vi "step7 SolveUpperRightCorner.vi"(11 "cube in":T1) -> (3 "cube out":T1)   [LabVIEW 2011]
uses:
  Typedef/cube.ctl
  Typedef/face.ctl
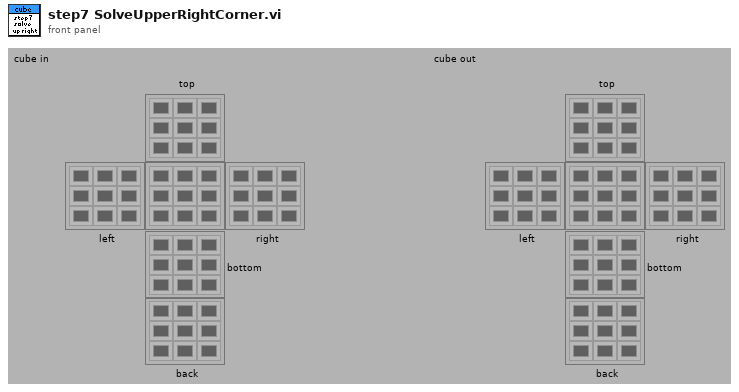
[diagram p1: front panel]
types:
  T1 = typedef "cube.ctl" = cluster{"top":T2, "left":T2, "right":T2, "bottom":T2, "back":T2, "front":T2}
  T2 = typedef "face.ctl" = u32[][]
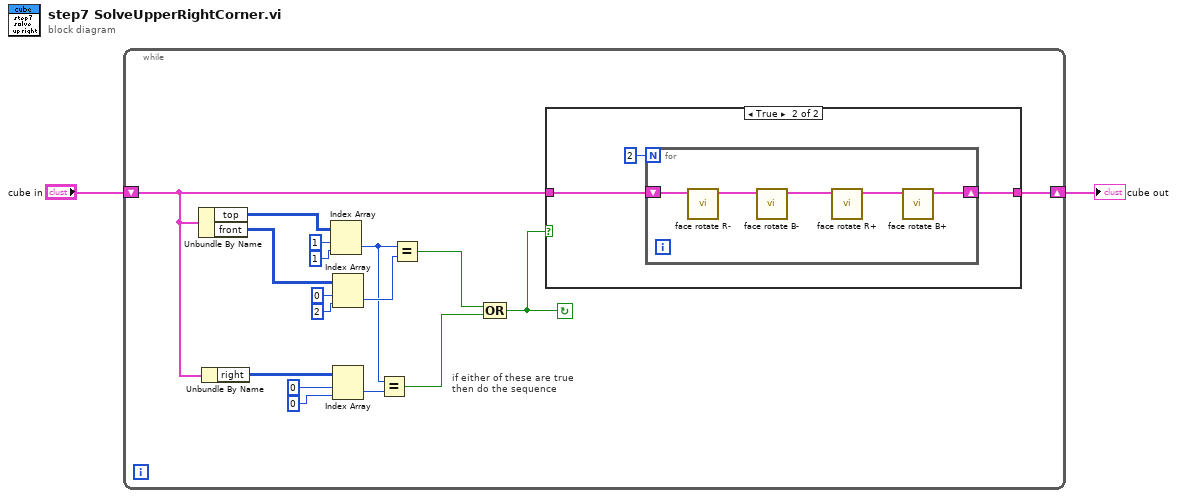
[diagram p0: block diagram]
diagram:
  n1 = while {
    shift-right: [w11] -> w1
    shift-left: "cube in" -> [w12]
    stop <- w10 continue-if-true
    # "if either of these are true\nthen do the sequence"
    n2 = Unbundle By Name(w12) -> ("top"=w9:T2, "front"=w6:T2)
    n3 = Unbundle By Name(w12) -> ("right"=w17:T2)
    n4 = Index Array(array=w9, index (row)=1, index (col)=1 ("disabled index (col)")) -> (element=w3:u32)
    n5 = Index Array(array=w6, index (row)=0, index (col)=2 ("disabled index (col)")) -> (element=w5:u32)
    n6 = Index Array(array=w17, index (row)=0, index (col)=0 ("disabled index (col)")) -> (element=w4:u32)
    n7 = Equal?(x=w3, y=w4) -> (x = y?=w13:bool)
    n8 = Equal?(x=w3, y=w5) -> (x = y?=w14:bool)
    n9 = Compound Arithmetic op=OR(w14, w13) -> (w10:bool)
    n10 = case shown="True" w10 {
      tunnel: w12 -> [w20 w23]
      tunnel: [w20 w22] -> w11
      frame False {
      }
      frame True {
        n11 = for {
          N: 2 -> [_]
          shift-right: [w24] -> w22
          shift-left: w23 -> [w28]
          n12 = call "face rotate R-.vi"("cube in"=w28) -> ("cube out"=w27:T1)  [unwired: 9 in, 1 out]
          n13 = call "face rotate B-.vi"("cube in"=w27) -> ("cube out"=w26:T1)  [unwired: 9 in, 1 out]
          n14 = call "face rotate R+.vi"("cube in"=w26) -> ("cube out"=w25:T1)  [unwired: 9 in, 1 out]
          n15 = call "face rotate B+.vi"("cube in"=w25) -> ("cube out"=w24:T1)  [unwired: 9 in, 1 out]
        }
      }
    }
  }
  "cube out" <- w1
